vi "col00.vi"(7 "error in (no error)":errorcluster) -> (21 "Col00 (B/AI0 (Pin 3))":dbl, 27 "error out":errorcluster)   [LabVIEW 2014]
doc: "Reads values from one or more analog input channels on the NI myRIO. Use this Express VI to read one or multiple samples for each channel at one time."
uses:
  <vilib>/myRIO/Common/Instrument Driver Framework/myRIO v1.0/AI/vis/myRIO v1.0 Read AI.vi
  <vilib>/Utility/error.llb/Error Cluster From Error Code.vi
  <vilib>/myRIO/Instrument Drivers/Onboard IO/AI/AI.lvlib
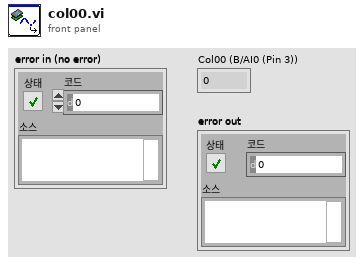
[diagram p1: front panel]
types:
  T1 = typedef "AI.lvlib/AI Reference.ctl" = cluster{"myRIO Reference":T2, "AI Channels List":T6, "AI Scaling Constants List":T8}
  T2 = typedef "myRIO Generic Hardware Reference.ctl" = cluster{"myRIO Model":T3, "myRIO Hardware Reference":T4}
  T3 = typedef "Hardware Version Enum.ctl" = enum16{"Unknown", "myRIO-1900", "myRIO-1950"}
  T4 = typedef "myRIO v1.0 Reference.ctl" = cluster{"Generic FPGA Reference":T5, "Allow multiple opens":bool}
  T5 = typedef "Generic FPGA Reference.ctl" = refnum<k20>
  T6 = typedef "AI Channels List.ctl" = T7[]
  T7 = typedef "AI Channels Enum.ctl" = enum16{"Not Connected", "AudioIn/Left", "AudioIn/Right", "C/AI0", "C/AI1", "A/AI0", "A/AI1", "A/AI2", "A/AI3", "B/AI0", "B/AI1", "B/AI2", "B/AI3"}
  T8 = typedef "Analog Scaling Constants List.ctl" = T9[]
  T9 = typedef "Analog Scaling Constants.ctl" = cluster{"LSB Weight (Volts)":dbl, "Offset (Volts)":dbl, "Signed?":bool}
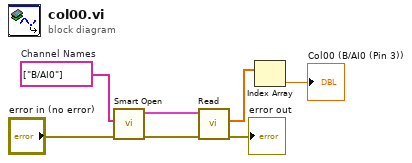
[diagram p0: block diagram]
diagram:
  w7 = tag[] ["B/AI0"]  # Channel Names
  n1 = call <vilib>:"Smart Open.vi"("error in (no error)"="error in (no error)", "Channel Names"=w7) -> ("error out"=w2:errorcluster, "AI Ref Out"=w3:T1)  [unwired: 8 in]
  n2 = call <vilib>:"Read.vi"("error in (no error)"=w2, "AI Ref In"=w3) -> ("error out"=→"error out":errorcluster, "Values"=w6:dbl[])  [unwired: 7 in, 1 out]
  n3 = Index Array(array=w6) -> (element=→"Col00 (B/AI0 (Pin 3))":dbl)  [unwired: 1 in]
